vi "Put_Array_into_String.vi"(1 "String array":string[](array[string])) -> (0 "String Value":string)   [LabVIEW 2010]
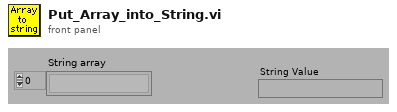
[diagram p1: front panel]
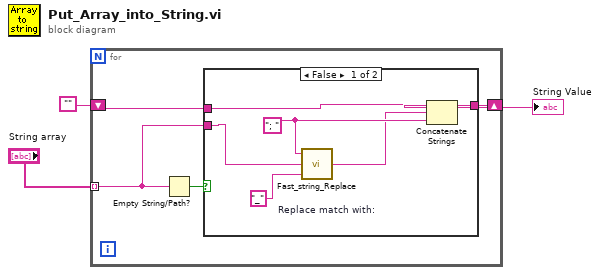
[diagram p0: block diagram]
diagram:
  n1 = for {
    shift-right: [w5] -> w1
    shift-left: "" -> [w6]
    tunnel: "String array" -> [w4] mode=indexing
    n2 = Empty String/Path?(string/path=w4) -> (empty?=w7:bool)
    n3 = case shown="False" w7 {
      tunnel: w6 -> [w13 w14]
      tunnel: [w12 w14] -> w5
      tunnel: w4 -> [w10 _]
      frame False {
        w9 = "_"  # Replace match with:
        w11 = "; " ("Substring")
        n4 = call "Fast_string_Replace.vi"("Replace match with:"=w9, "Input String"=w10, "regular expression"=w11) -> ("Output String"=w8:string)  [unwired: 2 out]
        n5 = Concatenate Strings(w13, w8, w11) -> (w12:string)
      }
      frame True {
      }
    }
  }
  "String Value" <- w1
